vi "Unit Delay (DBL).vi"(2 "initialize":bool, 3 "initial condition":dbl format="%.2f", 5 "input point":dbl format="%.2f") -> (1 "output point":dbl format="%.2f")   [LabVIEW 2020, in "NI_AdvCtrl_discrete linear.lvlib"]
doc: "LabVIEW no longer supports this VI. You can obtain similar functionality by installing the LabVIEW Simulation Module.\n\nDelays the input exactly one time step, i.e. output point[n]=input point[n-1], where output point[0]=initial condition."
uses:
  <vilib>/addons/control/advanced/NI_AdvCtrl_discrete linear.lvlib
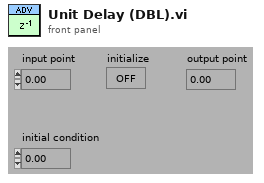
[diagram p1: front panel]
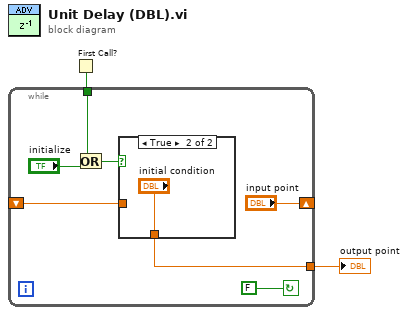
[diagram p0: block diagram]
diagram:
  n1 = First Call?() -> (First Call?: T/F=w1:bool)
  n2 = while {
    tunnel: w1 -> [w4]
    tunnel: [w8] -> w2
    shift-left: _ -> [w9]
    shift-right: ["input point"] -> _
    stop <- FALSE continue-if-true
    n3 = Or(x=w4, y="initialize") -> (x .or. y?=w6:bool)
    n4 = case shown="True" w6 {
      tunnel: [w10 "initial condition"] -> w8
      tunnel: w9 -> [w10 _]
      frame False {
      }
      frame True {
      }
    }
  }
  "output point" <- w2
